vi "droicam.vi"() -> ()   [LabVIEW 2020]
panel:
  out "Image Out":T1(plugin-control)
  in  "stop":bool
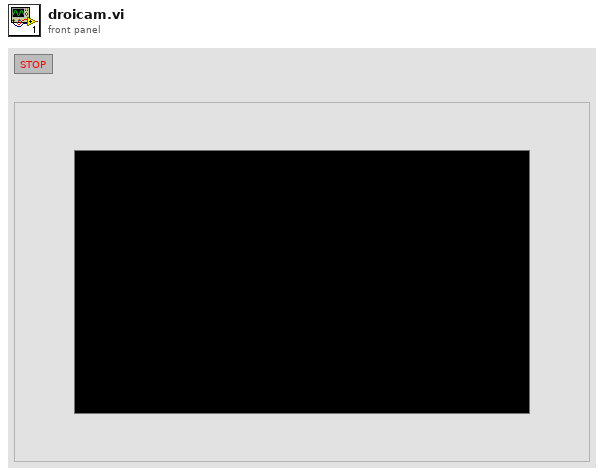
[diagram p1: front panel]
types:
  T1 = typedef "IMAQ Image.ctl" = refnum<image>
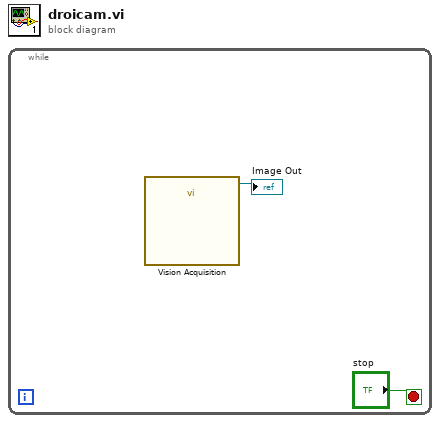
[diagram p0: block diagram]
diagram:
  n1 = while {
    stop <- "stop" stop-if-true
    n2 = call "Vision Acquisition"() -> ("Image Out"=→"Image Out":T1)  [unwired: 23 in, 4 out]
  }
